vi "CHS_ODOM_EXECUTE.vi"(6 "Pass_Through_Time":dbl=-1.0 format="%33.4f", 8 "error in (no error)":errorcluster) -> (0 "error out":errorcluster)   [LabVIEW 2019]
uses:
  <vilib>/Rock Robotics/WPI/ThirdParty/JAS_Junk/TrajLib/Rotation2d_Plus.vi
  <vilib>/Rock Robotics/WPI/ThirdParty/JAS_Junk/TrajLib/Twist2d_Create.vi
  <vilib>/Rock Robotics/WPI/ThirdParty/JAS_Junk/TrajLib/Rotation2d_Minus.vi
  <vilib>/Rock Robotics/WPI/ThirdParty/JAS_Junk/TrajLib/Pose2d_getTranslation.vi
  <vilib>/Rock Robotics/WPI/ThirdParty/JAS_Junk/TrajLib/Pose2d_New_TRRO.vi
  <vilib>/Rock Robotics/WPI/ThirdParty/JAS_Junk/TrajLib/VI/SwerveModulePosition_Get.vi
  <vilib>/Rock Robotics/WPI/ThirdParty/JAS_Junk/TrajLib/VI/SwerveModulePosition_New.vi
  <vilib>/Rock Robotics/WPI/ThirdParty/JAS_Junk/TrajLib/Twist2d_GetAll.vi
  <vilib>/Rock Robotics/WPI/ThirdParty/JAS_Junk/TrajLib/VI/Util_GetTime_U32.vi
  <vilib>/Rock Robotics/WPI/ThirdParty/JAS_Junk/TrajLib/Rotation2d_RotateBy.vi
  <vilib>/Rock Robotics/WPI/ThirdParty/JAS_Junk/TrajLib/Rotation2d_UnaryMinus.vi
  <vilib>/Rock Robotics/WPI/ThirdParty/JAS_Junk/TrajLib/Rotation2d_CreateXY.vi
  <vilib>/Rock Robotics/WPI/ThirdParty/JAS_Junk/TrajLib/Util_CalcDist.vi
  CHS_ODOM_GLOBALS.vi
  Swerve_Drive_System/CHS_DRIVE_GLOBALS.vi
  <vilib>/Rock Robotics/WPI/ThirdParty/JAS_Junk/TrajLib/VI/SwerveKinematics_ToTwist2dX.vi
  <vilib>/Rock Robotics/WPI/ThirdParty/JAS_Junk/TrajLib/Pose2d_Exp.vi
  <vilib>/Rock Robotics/WPI/ThirdParty/JAS_Junk/TrajLib/VI/Util_GetTime_U64.vi
  <vilib>/Rock Robotics/WPI/ThirdParty/JAS_Junk/TrajLib/Trajectory_Library.lvlib
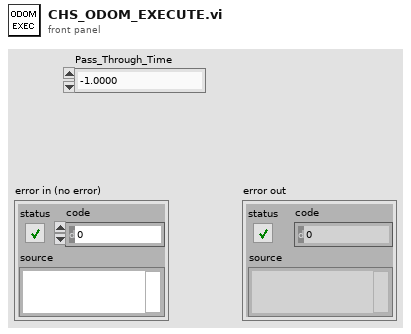
[diagram p1: front panel]
types:
  T1 = typedef "Trajectory_Library.lvlib/SWERVE_DRIVE_KINEMATICS.ctl" = cluster{"NumModules":i32, "InverseKinematics":T2, "ForwardKinematics":T2, "Modules":T3[], "PrevCoR":T3, "SavedModuleStates":T4[]}
  T2 = typedef "NI_Matrix.lvlib/RealMatrix.ctl" = dbl[][]
  T3 = typedef "Trajectory_Library.lvlib/TRANSLATION2D.ctl" = cluster{"X":dbl, "Y":dbl}
  T4 = typedef "Trajectory_Library.lvlib/SWERVE_DRIVE_MODULE_STATE.ctl" = cluster{"Speed":dbl, "Angle":T5}
  T5 = typedef "Trajectory_Library.lvlib/ROTATION2D.ctl" = cluster{"VALUE":dbl, "COS":dbl, "SIN":dbl}
  T6 = typedef "Trajectory_Library.lvlib/SWERVE_DRIVE_ODOMETRY.ctl" = cluster{"POSE":T7, "GyroOffset":T5, "PreviousAngle":T5, "PrevModulePositions":T8[], "NumModules":i32}
  T7 = typedef "Trajectory_Library.lvlib/POSE2D.ctl" = cluster{"TRANSLATION":T3, "ROTATION":T5}
  T8 = typedef "Trajectory_Library.lvlib/SWERVE_DRIVE_MODULE_POSITION.ctl" = cluster{"Distance":dbl, "Angle":T5, "P":bool}
  T9 = typedef "Trajectory_Library.lvlib/SWERVE_DRIVE_POSE_EST2_CONFIG.ctl" = cluster{"Wheel_Locations M":T3[], "Odom X std dev M":dbl, "Odom Y std dev M":dbl, "Odom Heading std dev Rad":dbl, "Vision X std dev M":dbl, "Vision Y std dev M":dbl, "Vision Heading std dev Rad":dbl}
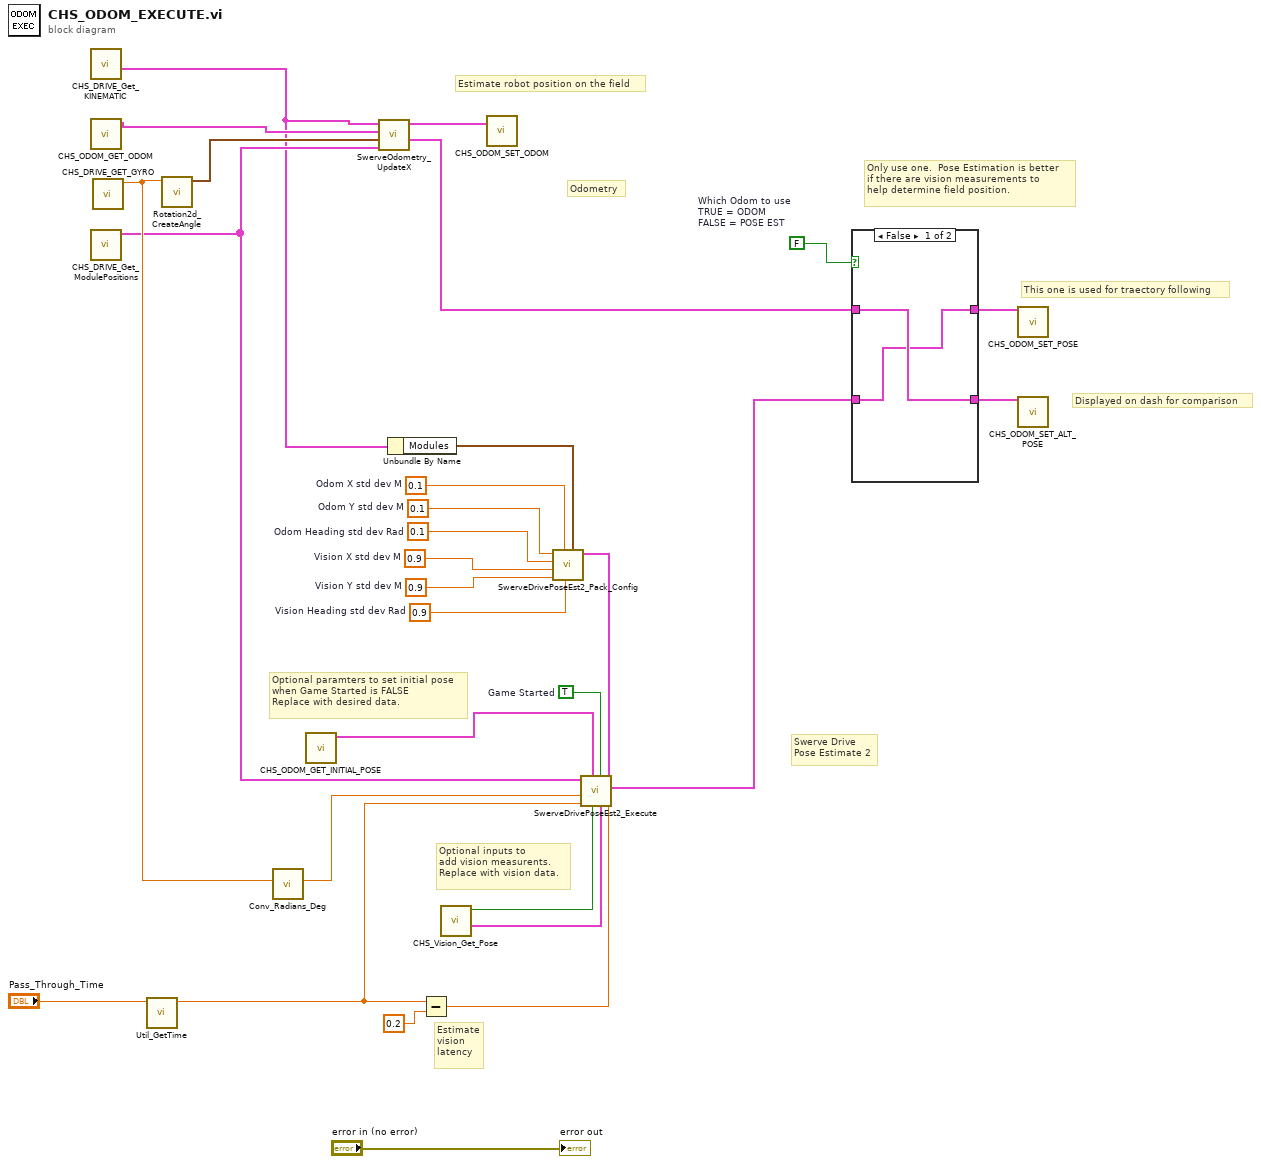
[diagram p0: block diagram]
diagram:
  w5 = 0.1  # Odom Y std dev M
  w6 = 0.1  # Odom Heading std dev Rad
  w7 = 0.9  # Vision X std dev M
  w8 = 0.9  # Vision Y std dev M
  w9 = 0.1  # Odom X std dev M
  w10 = 0.9  # Vision Heading std dev Rad
  w26 = FALSE  # Which Odom to use TRUE = ODOM FALSE = POSE EST
  w18 = TRUE  # Game Started
  # "Displayed on dash for comparison"
  # "Estimate\nvision \nlatency"
  # "This one is used for traectory following"
  # "Only use one.  Pose Estimation is better\nif there are vision measurements to\nhelp determine field position."
  # "Optional inputs to\nadd vision measurents.\nReplace with vision data."
  # "Optional paramters to set initial pose\nwhen Game Started is FALSE\nReplace with desired data."
  # "Swerve Drive \nPose Estimate 2"
  # "Odometry"
  # "Estimate robot position on the field"
  n1 = call "CHS_DRIVE_Get_KINEMATIC.vi"() -> ("out SWERVE_DRIVE_KINEMATICS"=w2:T1)  [unwired: 11 in]
  n2 = call "CHS_ODOM_GET_ODOM.vi"() -> ("Absolue Odometry"=w3:T6)  [unwired: 11 in]
  n3 = call "CHS_DRIVE_Get_ModulePositions.vi"() -> ("Swerve Module Positions"=w15:T8[])  [unwired: 11 in]
  n4 = call "CHS_DRIVE_GET_GYRO.vi"() -> ("Gyro Heading Radians"=w23:dbl)  [unwired: 11 in]
  n5 = call <vilib>:"Util_GetTime.vi"("Pass_Through_Time"="Pass_Through_Time") -> ("FPGA_Time_Seconds"=w12:dbl)  [unwired: 8 in, 2 out]
  n6 = call <vilib>:"Rotation2d_CreateAngle.vi"("Angle"=w23) -> ("ROTATION"=w22:T5)  [unwired: 10 in]
  n7 = call <vilib>:"Conv_Radians_Deg.vi"("Radians"=w23) -> ("Degrees"=w14:dbl)  [unwired: 10 in]
  n8 = call "CHS_ODOM_GET_INITIAL_POSE.vi"() -> ("Initial Odometry Pose"=w19:T7)  [unwired: 11 in]
  n9 = call <vilib>:"SwerveOdometry_UpdateX.vi"("module Positions"=w15, "gyroAngle"=w22, "in SWERVE_DRIVE_ODOMETRY"=w3, "SWERVE_DRIVE_KINEMATICS"=w2) -> ("robot POSE"=w20:T7, "out SWERVE_DRIVE_ODOMETRY"=w21:T6)  [unwired: 5 in, 1 out]
  n10 = Unbundle By Name(w2) -> ("Modules"=w1:T3[])
  n11 = Subtract(x=w12, y=0.2) -> (x-y=w13:dbl)
  n12 = call "CHS_Vision_Get_Pose.vi"() -> ("Vison Pose"=w17:T7, "Have Vision Pose"=w16:bool)  [unwired: 10 in]
  n13 = call "CHS_ODOM_SET_ODOM.vi"("Absolue Odometry"=w21) -> ()  [unwired: 11 in]
  n14 = call <vilib>:"SwerveDrivePoseEst2_Pack_Config.vi"("Wheel_Locations M"=w1, "Vision Heading std dev Rad"=w10, "Odom X std dev M"=w9, "Vision Y std dev M"=w8, "Vision X std dev M"=w7, "Odom Heading std dev Rad"=w6, "Odom Y std dev M"=w5) -> ("SwervePoseEst2Config"=w4:T9)  [unwired: 4 in]
  n15 = call <vilib>:"SwerveDrivePoseEst2_Execute.vi"("Vision TImeStamp_Seconds"=w13, "SwervePoseEst2Config"=w4, "visionRobotPose"=w17, "Game Started"=w18, "Add Vision Meas"=w16, "InitialPose"=w19, "Pass Through Time"=w12, "Gyro Degrees"=w14, "Module Positions"=w15) -> ("Estimated Pose"=w11:T7)  [unwired: 1 in, 1 out]
  n16 = case shown="False" w26 {
    tunnel: w20 -> [w31 w33]
    tunnel: [w30 w33] -> w27
    tunnel: w11 -> [w30 w32]
    tunnel: [w31 w32] -> w24
    frame False {
    }
    frame True {
    }
  }
  n17 = call "CHS_ODOM_SET_POSE.vi"("Absolute Odometry Pose"=w27) -> ()  [unwired: 11 in]
  n18 = call "CHS_ODOM_SET_ALT_POSE.vi"("Odometry ALT Pose"=w24) -> ()  [unwired: 11 in]
  "error out" <- "error in (no error)"
